vi "ClsLastError.vi"(8 "error in (no error)":errorcluster) -> (0 "error out":errorcluster, 3 "Error Message":string)   [LabVIEW 2015]
doc: "Last Error:\n\nCall this function if any of the DLL functions return an error code to obtain an error message. Should be used within the provided subVIs and not by the user directly.\n\nError Message[Output]: the error message indicating the error."
uses:
  dependent dlls/CHRocodileDLL.dll
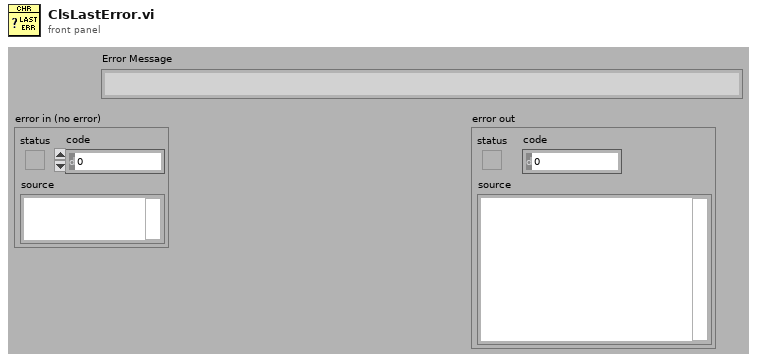
[diagram p1: front panel]
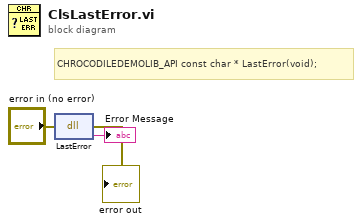
[diagram p0: block diagram]
diagram:
  # "CHROCODILEDEMOLIB_API const char * LastError(void);"
  n1 = dll-call lib="C:/Users/privat/Documents/ADP-SLA/Drop Impact Teststand/dependent dlls/CHRocodileDLL.dll" fn="LastError"(error in="error in (no error)") -> (error out=→"error out":errorcluster, "return type"=→"Error Message":string)  [unwired: 2 in, 1 out]
